vi "GEOM_GetTofFPASize.vi"(10 "Correctedamplifier":T1, 11 "Database RefNum in":T2) -> (1 "Correctedamplifier out":T1, 2 "fpasize":string)   [LabVIEW 2016]
uses:
  GEOM_CorrectedFPA.ctl
  DBSHAND/private/vis/DatabaseHand_RefNum.ctl
  GEOM_VAR_action.ctl
  DBSHAND/private/vis/DatabaseHand_Element_Get(string).vi
  DBSHAND/private/vis/DatabaseHand_Element_Set(string).vi
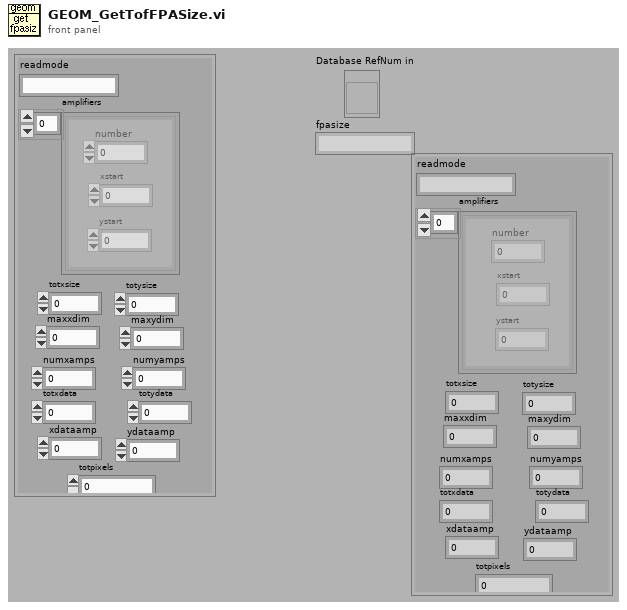
[diagram p1: front panel]
types:
  T1 = typedef "GEOM_CorrectedFPA.ctl" = cluster{"readmode":string, "amplifiers":cluster{"number":i32, "xstart":i32, "ystart":i32}[], "totxsize":i32, "totysize":i32, "maxxdim":i32, "maxydim":i32, "numxamps":i32, "numyamps":i32, "totxdata":i32, "totydata":i32, "xdataamp":i32, "ydataamp":i32, "totpixels":i32}
  T2 = typedef "DatabaseHand_RefNum.ctl" = refnum<vi>
  T3 = typedef "GEOM_VAR_action.ctl" = enum16{"read", "write"}
  T4 = typedef "GEOM_CoordsRef.ctl" = cluster{"xref":u32, "yref":u32}
  T5 = typedef "GEOM_DetSummaryStruct.ctl" = cluster{"detxpos":i32, "detypos":i32, "cols":i32, "rows":i32, "nxamps":i32, "nyamps":i32, "number":i32, "discard":i32, "totcols":i32, "totrows":i32, "readmode":string}
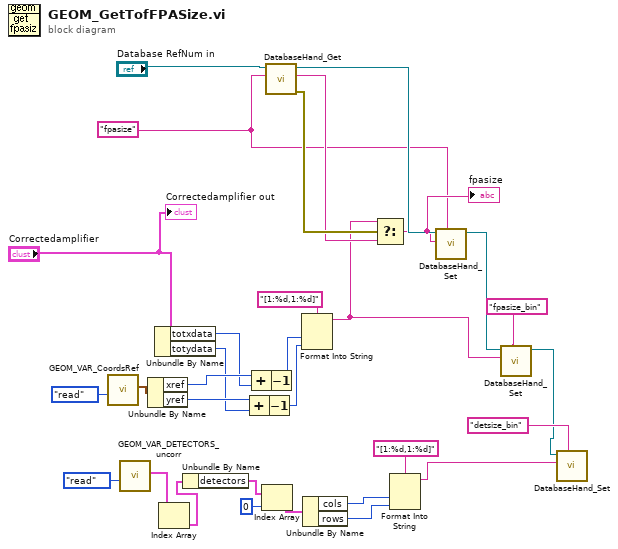
[diagram p0: block diagram]
diagram:
  w16 = "fpasize" ("name")
  n1 = call "GEOM_VAR_CoordsRef.vi"("Action"=GEOM_VAR_action."read") -> ("GEOM_coordsref out"=w31:T4)  [unwired: 1 in, 9 out]
  n2 = call "GEOM_VAR_DETECTORS_uncorr.vi"("Action"=GEOM_VAR_action."read") -> ("det out"=w3:cluster{"name":string, "detectors":T5[]}[])  [unwired: 1 in, 9 out]
  n3 = Unbundle By Name(w31) -> ("xref"=w30:u32, "yref"=w29:u32)
  n4 = Unbundle By Name("Correctedamplifier") -> ("totxdata"=w28:i32, "totydata"=w27:i32)
  n5 = Index Array(array=w3) -> (element=w2:cluster{"name":string, "detectors":T5[]})  [unwired: 1 in]
  n6 = Unbundle By Name(w2) -> ("detectors"=w9:T5[])
  n7 = Add(x=w29, y=w27) -> (x+y=w25:u32)
  n8 = Add(x=w30, y=w28) -> (x+y=w26:u32)
  n9 = Index Array(array=w9, index=0) -> (element=w7:T5)
  n10 = Decrement(x=w25) -> (x-1=w23:u32)
  n11 = call-poly "DatabaseHand_Get.vi"("name"=w16, "Database RefNum in"="Database RefNum in") -> ("error out"=w22:errorcluster, "value"=w21:string, "Database RefNum out"=w19:T2)  [unwired: 3 in, 4 out]
  n12 = Decrement(x=w26) -> (x-1=w24:u32)
  n13 = Format Into String(format string="[1:%d,1:%d]", w24, w23) -> (resulting string=w14:string)  [unwired: 2 in, 1 out]
  n14 = Unbundle By Name(w7) -> ("cols"=w6:i32, "rows"=w5:i32)
  n15 = Select(t=w14, s=w22, f=w21) -> (s? t:f=w18:string)
  "fpasize" <- w18
  n16 = Format Into String(format string="[1:%d,1:%d]", w6, w5) -> (resulting string=w10:string)  [unwired: 2 in, 1 out]
  n17 = call-poly "DatabaseHand_Set.vi"("name"=w16, "value"=w18, "Database RefNum in"=w19) -> ("Database RefNum out"=w15:T2)  [unwired: 5 in, 3 out]
  n18 = call-poly "DatabaseHand_Set.vi"("name"="fpasize_bin", "value"=w14, "Database RefNum in"=w15) -> ("Database RefNum out"=w1:T2)  [unwired: 5 in, 3 out]
  n19 = call-poly "DatabaseHand_Set.vi"("name"="detsize_bin", "value"=w10, "Database RefNum in"=w1) -> ()  [unwired: 5 in, 4 out]
  "Correctedamplifier out" <- "Correctedamplifier"
